vi "AKD Set Torque.vi"(0 "connection ID":refnum<k5>, 5 "Target torque (%+/-1000)":i32, 7 "Motor IPeak":sgl, 11 "error in":errorcluster) -> (4 "TCP Refnum":refnum<k5>, 15 "error out":errorcluster)   [LabVIEW 2019]
uses:
  MODBUS/NI Modbus.llb/MB Ethernet Master Query Write Multiple Registers (poly).vi
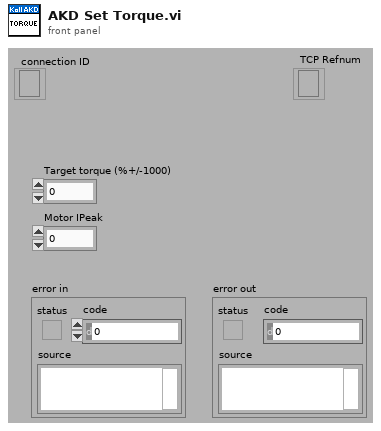
[diagram p1: front panel]
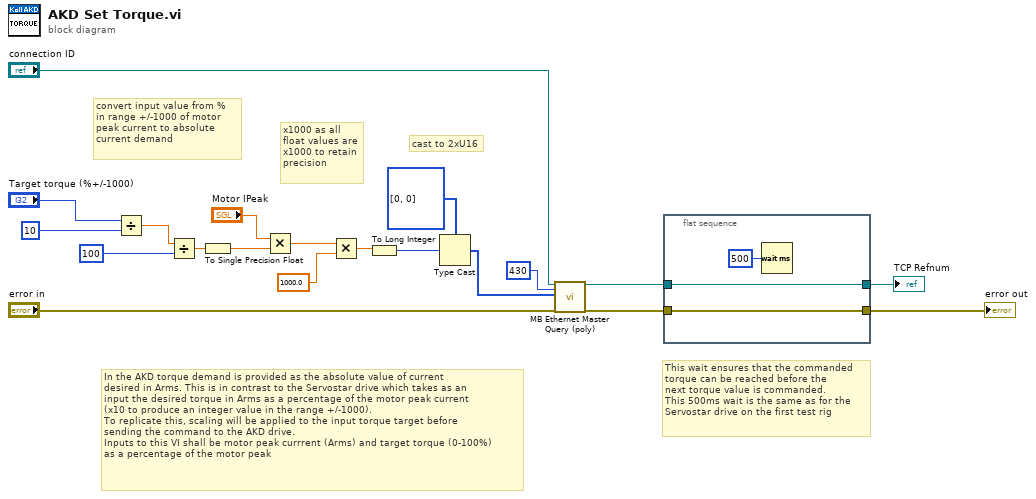
[diagram p0: block diagram]
diagram:
  # "This wait ensures that the commanded\ntorque can be reached before the\nnext torque value is commanded.\nThis 500ms wait is the same as for the\nServostar drive on the first test rig"
  # "cast to 2xU16"
  # "x1000 as all\nfloat values are\nx1000 to retain\nprecision"
  # "convert input value from %\nin range +/-1000 of motor\npeak current to absolute\ncurrent demand"
  # "In the AKD torque demand is provided as the absolute value of current\ndesired in Arms. This is in contrast to the Servostar drive which takes as an \ninput the desired torque in Arms as a percentage of the motor peak current\n(x10 to produce an integer value in the range +/-1000).\nTo replicate this, scaling will be applied to the input torque target before\nsending the command to the AKD drive.\nInputs to this VI shall be motor peak currrent (Arms) and target torque (0-100%)\nas a percentage of the motor peak"
  n1 = Divide(x="Target torque (%+/-1000)", y=10) -> (x/y=w16:dbl)
  n2 = Divide(x=w16, y=100) -> (x/y=w14:dbl)
  n3 = To Single Precision Float(number=w14) -> (single precision float=w6:sgl)
  n4 = Multiply(x="Motor IPeak", y=w6) -> (x*y=w7:sgl)
  n5 = Multiply(x=w7, y=sgl 1000.0) -> (x*y=w10:sgl)
  n6 = To Long Integer(number=w10) -> (32bit integer=w9:i32)
  n7 = Type Cast(type=u16[] [0, 0] ("Holding Registers"), x=w9) -> (*(type *) &x=w5:u16[])
  n8 = call-poly "MB Ethernet Master Query (poly).vi"("TCP Connection Refnum in"="connection ID", "Starting Address"=u16 430, "Registers"=w5, "error in"="error in") -> ("TCP Connection Refnum (dup)"=w1:refnum<k5>, "error out"=w3:errorcluster)  [unwired: 13 in, 1 out]
  n9 = flat-sequence {
    tunnel: [w22] -> w4
    tunnel: w3 -> [w22]
    tunnel: [w21] -> w2
    tunnel: w1 -> [w21]
    frame #0 {
      n10 = Wait (ms)(milliseconds to wait=u32 500) -> ()  [unwired: 1 out]
    }
  }
  "error out" <- w4
  "TCP Refnum" <- w2
